vi "Inst.RP100.setState.vi"(8 "error in (no error)":errorcluster, 10 "data in":variant, 11 "Inst.RP100 in":refnum<class "Inst.RP100.lvclass">) -> (0 "error out":errorcluster, 3 "Inst.RP100 out":refnum<class "Inst.RP100.lvclass">)   [LabVIEW 2019, in "Inst.RP100.lvlib" / "Inst.RP100.lvclass"]
uses:
  Inst.RP100.lvclass
  Typedefs/Channel--Num.ctl
  Typedefs/setState--Cluster.ctl
  Typedefs/State--Enum.ctl
  Inst.RP100.lvclass/Inst.RP100.ctl
  33339d53-136a-42ea-83c3-21456eeb2dd6.vi
  33339d53-136a-42ea-83c3-21456eeb2dd6.vi/f698b68b-f297-4516-9760-8926def79ee7.vi
  33339d53-136a-42ea-83c3-21456eeb2dd6.vi/7b657777-89be-4e60-a1bf-9fef44e7d3e5.vi
  <vilib>/Utility/Data Type/Get Type Information.vi
  <vilib>/JDP Science/JSONtext/JSON text to Variant.vi
  <vilib>/JDP Science/JSONtext/LVClass Serializer/JSONtext LVClass Serializer.lvclass
  RP100/RP100.lvlib
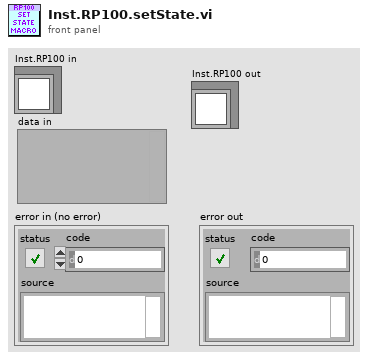
[diagram p1: front panel]
types:
  T1 = typedef "Inst.RP100.lvlib/Inst.RP100.lvclass/setState--Cluster.ctl" = cluster{"State":T2}
  T2 = typedef "Inst.RP100.lvlib/Inst.RP100.lvclass/State--Enum.ctl" = enum16{"Shorted", "Enabled"}
  T3 = typedef "Inst.RP100.lvlib/Inst.RP100.lvclass/Channel--Num.ctl" = i32
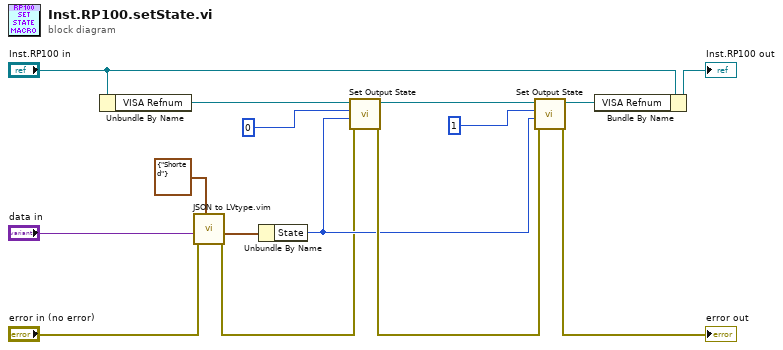
[diagram p0: block diagram]
diagram:
  n1 = Unbundle By Name("Inst.RP100 in") -> ("VISA Refnum"=w9:refnum<visa-resource-name>)
  n2 = call "JSON to LVtype.vim"("type"=T1 {"State"=enum."Shorted"} ("Data out"), "error in (no error)"="error in (no error)", "JSON Data in"="data in") -> ("error out"=w1:errorcluster, "Data out"=w4:T1)  [unwired: 7 in]
  n3 = Unbundle By Name(w4) -> ("State"=w10:T2)
  n4 = call "Set Output State.vi"("error in (no error)"=w1, "Output State"=w10, "Output Channel"=T3 0, "VISA resource name"=w9) -> ("error out"=w14:errorcluster, "VISA Refnum out"=w13:refnum<visa-resource-name>)  [unwired: 5 in, 1 out]
  n5 = call "Set Output State.vi"("error in (no error)"=w14, "Output State"=w10, "Output Channel"=T3 1, "VISA resource name"=w13) -> ("error out"=→"error out":errorcluster, "VISA Refnum out"=w8:refnum<visa-resource-name>)  [unwired: 5 in, 1 out]
  n6 = Bundle By Name(cluster="Inst.RP100 in", "VISA Refnum"=w8) -> (→"Inst.RP100 out":refnum<class "Inst.RP100.lvclass">)
